vi "Destroy.vi"(8 "error in (no error)":errorcluster, 11 "Select In":refnum<class "Select.lvclass">) -> (0 "error out":errorcluster, 3 "Select Out":refnum<class "Select.lvclass">)   [LabVIEW 2017, in "Front Panel Publisher.lvlib" / "Select.lvclass"]
uses:
  Select.lvclass
  Control_class/Control.lvclass
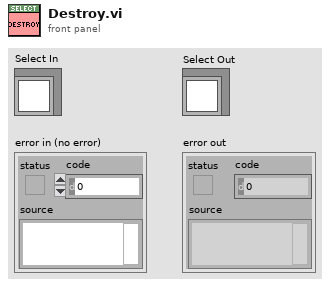
[diagram p1: front panel]
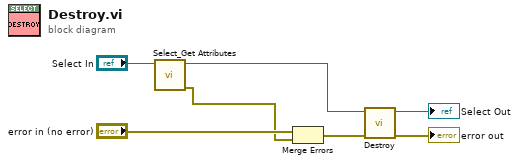
[diagram p0: block diagram]
diagram:
  n1 = call "Select_Get Attributes.vi"("Select In"="Select In") -> ("error out"=w1:errorcluster, "Select Out"=w5:refnum<class "Select.lvclass">)  [unwired: 8 in, 1 out]
  n2 = Merge Errors("error in (no error)", w1) -> (w3:errorcluster)
  n3 = call-parent "Destroy.vi"("error in (no error)"=w3, "Control In"=w5) -> ("error out"=→"error out":errorcluster, "Control Out"=→"Select Out":refnum<class "Select.lvclass">)  [unwired: 8 in]
